vi "Finalize.vi"(2 "error in (no error)":errorcluster) -> (0 "error out":errorcluster, 1 "Enum":T1(ring)=enum."Initialize")   [LabVIEW 2017]
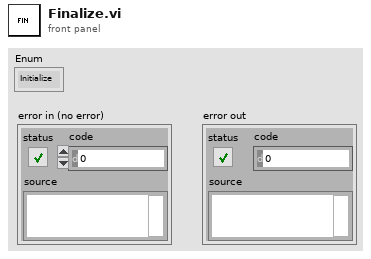
[diagram p1: front panel]
types:
  T1 = enum16{"Terminate", "Finalize", "Execute", "Initialize"}
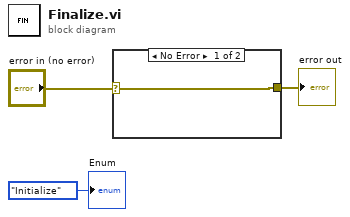
[diagram p0: block diagram]
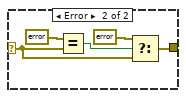
[diagram p2: hidden frame]
diagram:
  n1 = case shown="No Error" "error in (no error)" {
    selector: "error in (no error)" -> [w4 w6]
    tunnel: [w4 w7] -> w3
    frame No Error {
    }
    frame Error {
      n2 = Equal?(x=errorcluster {"status"=TRUE, "code"=80085, "source"="Terminated From App"} ("error out"), y=w6) -> (x = y?=w9:bool)
      n3 = Select(t=errorcluster {"status"=FALSE, "code"=80085, "source"="Terminated from App"} ("error in (no error)"), s=w9, f=w6) -> (s? t:f=w7:errorcluster)
    }
  }
  "error out" <- w3
  "Enum" <- T1."Initialize"
